vi "hyst_sat_drift_cascade_parallel_debug.vi"(4 "N_hyst":i32, 5 "reset":bool, 6 "N_sat":i32, 8 "Den":sgl[](array[numeric])=[0.982758, -1.98194, 1.0, 0.0, 0.0, 0.0, 0.0, 0.0, 0.0], 9 "Num":sgl[](array[numeric])=[-0.00254, 0.000408, 0.00295, 0.0, 0.0, 0.0, 0.0, 0.0, 0.0], 10 "TF Order":i32=2, 11 "u_k (un saturated)":fxp<+/-,16,5>) -> (2 "Hinv(uk)":fxp<+/-,32,10>)   [LabVIEW 2017]
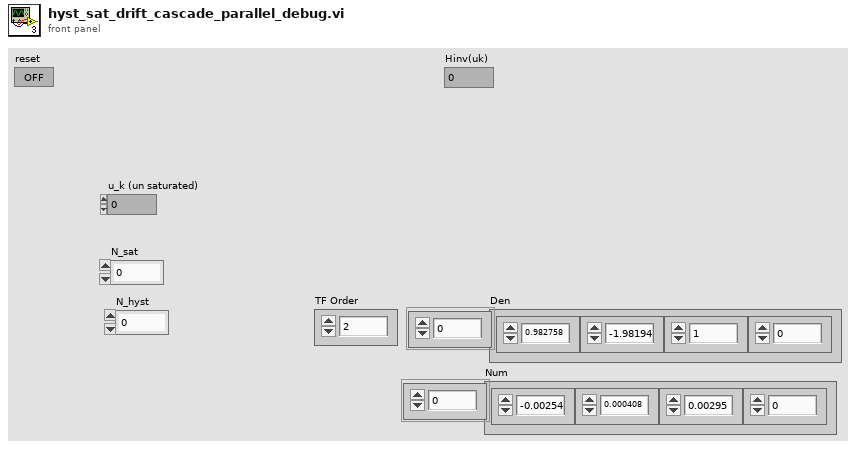
[diagram p1: front panel]
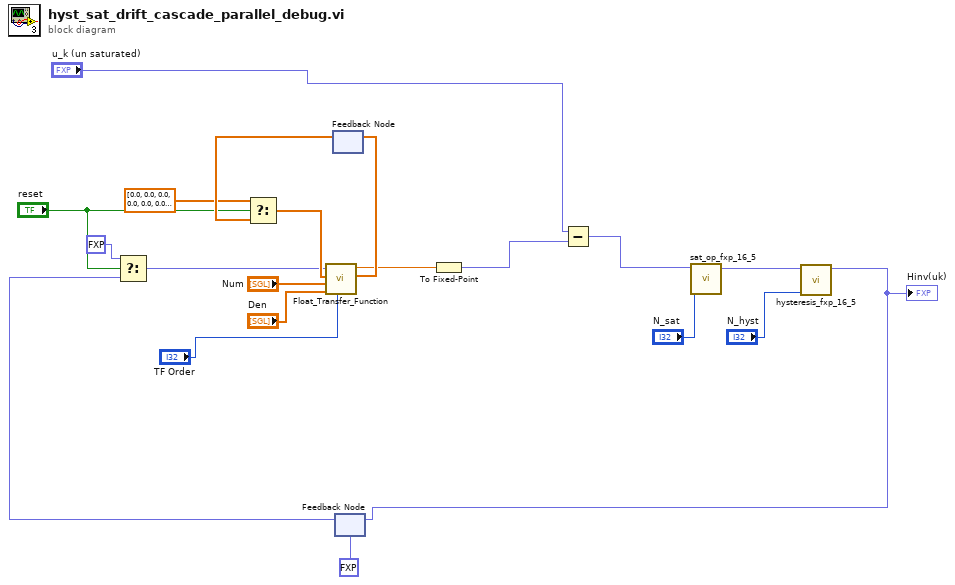
[diagram p0: block diagram]
diagram:
  n1 = feedback #1() -> (w12:sgl[])  [unwired: 1 in]
  n2 = Select(t=sgl[] [0.0, 0.0, 0.0, 0.0, 0.0, 0.0, 0.0, 0.0, 0.0] ("State Out"), s="reset", f=w12) -> (s? t:f=w11:sgl[])
  n3 = feedback #2(fxp<+/-,32,10> 0.0 ("Hinv(uk)")) -> (w8:fxp<+/-,32,10>)
  n4 = Select(t=fxp<+/-,32,10> 0.0, s="reset", f=w8) -> (s? t:f=w5:fxp<+/-,32,10>)
  n5 = call "Float_Transfer_Function.vi"("TF Order"="TF Order", "Den"="Den", "Num"="Num", "State In"=w11, "Input"=w5) -> ("State Out"=w16:sgl[], "Output"=w4:sgl)  [unwired: 4 in]
  n6 = feedback-in #1(w16) -> ()
  n7 = To Fixed-Point(number=w4) -> (fixed-point=w3:fxp<+/-,16,5>)  [unwired: 1 in]
  n8 = Subtract(x="u_k (un saturated)", y=w3) -> (x-y=w2:fxp<+/-,16,5>)
  n9 = call "sat_op_fxp_16_5.vi"("N_sat"="N_sat", "uk_in"=w2) -> ("Hinv(uk)"=w20:fxp<+/-,32,10>)  [unwired: 9 in]
  n10 = call "hysteresis_fxp_16_5.vi"("N_hyst"="N_hyst", "uk_in"=w20) -> ("Hinv(uk)"=w1:fxp<+/-,32,10>)  [unwired: 9 in]
  "Hinv(uk)" <- w1
  n11 = feedback-in #2(w1) -> ()
